vi "Query Registers.vi"(0 "VISA Resource Name":refnum<visa-resource-name>, 5 "Reg (11:dq STATUS GROUP: EVENT)":T1(ring)=enum."dq STATUS GROUP: EVENT", 11 "error in (no error)":errorcluster {"code" format="%.0x"}) -> (4 "VISA Resource Name Out":refnum<visa-resource-name>, 6 "Register Data":string, 15 "error out":errorcluster {"code" format="%.0x"})   [LabVIEW 2012, in "Agilent ESG Series.lvlib"]
doc: "This VI is used query the instrument about various operational and tracking data."
uses:
  <instrlib>/Agilent ESG Series/Agilent ESG Series.lvlib
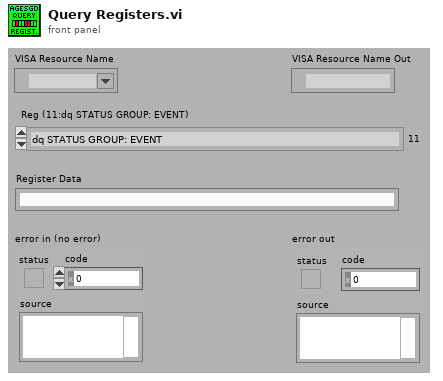
[diagram p1: front panel]
types:
  T1 = enum16{"dq BERT STATUS GROUP: CONDITION", "dq BERT STATUS GROUP: EVENT", "dq CALIBRATION STATUS GROUP: CONDITION", "dq CALIBRATION STATUS GROUP: EVENT", "dq FREQUENCY STATUS GROUP: CONDITION", "dq FREQUENCY STATUS GROUP: EVENT", "dq MODULATION STATUS GROUP: CONDITION", "dq MODULATION STATUS GROUP: EVENT", "dq POWER STATUS GROUP: CONDITION", "dq POWER STATUS GROUP: EVENT", "dq STATUS GROUP: CONDITION", "dq STATUS GROUP: EVENT", "so STATUS GROUP: CONDITION", "so STATUS GROUP: EVENT"}
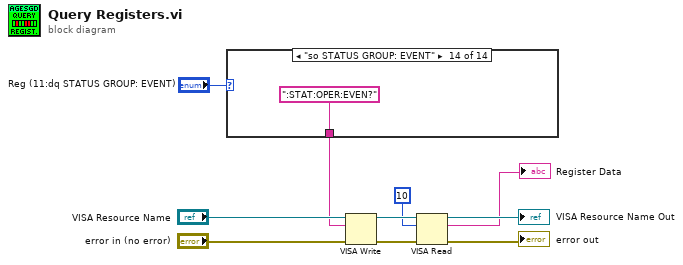
[diagram p0: block diagram]
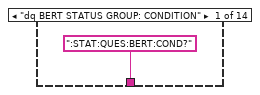
[diagram p2: hidden frame]
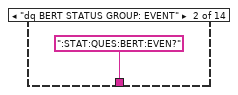
[diagram p3: hidden frame]
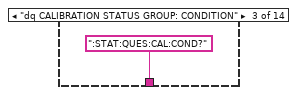
[diagram p4: hidden frame]
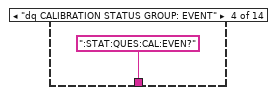
[diagram p5: hidden frame]
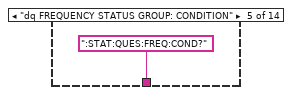
[diagram p6: hidden frame]
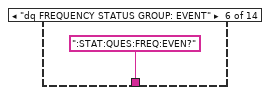
[diagram p7: hidden frame]
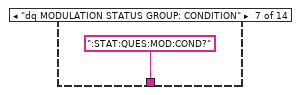
[diagram p8: hidden frame]
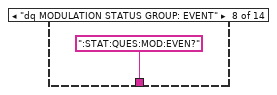
[diagram p9: hidden frame]
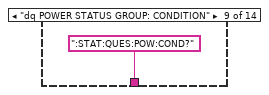
[diagram p10: hidden frame]
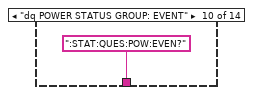
[diagram p11: hidden frame]
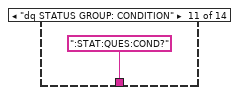
[diagram p12: hidden frame]
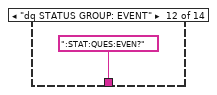
[diagram p13: hidden frame]
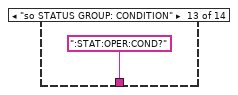
[diagram p14: hidden frame]
diagram:
  n1 = case shown="\"so STATUS GROUP: EVENT\"" "Reg (11:dq STATUS GROUP: EVENT)" {
    tunnel: [":STAT:QUES:BERT:COND?" ":STAT:QUES:BERT:EVEN?" ":STAT:QUES:CAL:COND?" ":STAT:QUES:CAL:EVEN?" ":STAT:QUES:FREQ:COND?" ":STAT:QUES:FREQ:EVEN?" ":STAT:QUES:MOD:COND?" ":STAT:QUES:MOD:EVEN?" ":STAT:QUES:POW:COND?" ":STAT:QUES:POW:EVEN?" ":STAT:QUES:COND?" ":STAT:QUES:EVEN?" ":STAT:OPER:COND?" ":STAT:OPER:EVEN?"] -> w8
    frame "dq BERT STATUS GROUP: CONDITION" {
    }
    frame "dq BERT STATUS GROUP: EVENT" {
    }
    frame "dq CALIBRATION STATUS GROUP: CONDITION" {
    }
    frame "dq CALIBRATION STATUS GROUP: EVENT" {
    }
    frame "dq FREQUENCY STATUS GROUP: CONDITION" {
    }
    frame "dq FREQUENCY STATUS GROUP: EVENT" {
    }
    frame "dq MODULATION STATUS GROUP: CONDITION" {
    }
    frame "dq MODULATION STATUS GROUP: EVENT" {
    }
    frame "dq POWER STATUS GROUP: CONDITION" {
    }
    frame "dq POWER STATUS GROUP: EVENT" {
    }
    frame "dq STATUS GROUP: CONDITION" {
    }
    frame "dq STATUS GROUP: EVENT" {
    }
    frame "so STATUS GROUP: CONDITION" {
    }
    frame "so STATUS GROUP: EVENT" {
    }
  }
  n2 = VISA Write(VISA resource name="VISA Resource Name", write buffer=w8, error in (no error)="error in (no error)") -> (VISA resource name out=w7:refnum<visa-resource-name>, error out=w6:errorcluster)  [unwired: 1 out]
  n3 = VISA Read(VISA resource name=w7, byte count=u32 10 ("byte count (0)"), error in (no error)=w6) -> (VISA resource name out=→"VISA Resource Name Out":refnum<visa-resource-name>, read buffer=→"Register Data":string, error out=→"error out":errorcluster)  [unwired: 1 out]
